vi "Actor Core.vi"(8 "error in":errorcluster, 11 "Microscope in":refnum<class "Microscope.lvclass">) -> (0 "error out":errorcluster, 3 "Actor out":refnum<class "Actor.lvclass">)   [LabVIEW 2020, in "Microscope.lvlib" / "Microscope.lvclass"]
doc: "(<B>Filename</B>: Actor Framework.lvlib:Actor.lvclass:Actor Core.vi)\n\nReceives messages to the actor, reacts to them, and initiates any error handling that may shut the actor down.\n\nDescendant classes may override this VI to append parallel tasks for the actor to complete while it handles messages. Overrides use the Call Parent Class Method node."
uses:
  Microscope.lvclass
  C:/Program Files/National Instruments/LabVIEW 2020/vi.lib/ActorFramework/Actor/Actor.lvclass
  <vilib>/ActorFramework/Actor/Actor.lvclass
  Microscope Controller/Microscope Controller.lvclass
  Microscope.lvclass/Microscope.ctl
  Device/Device/Device.lvclass
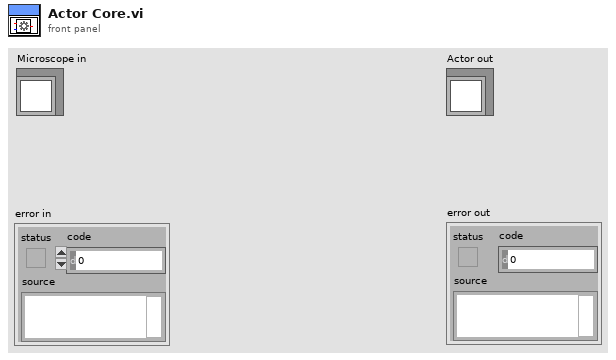
[diagram p1: front panel]
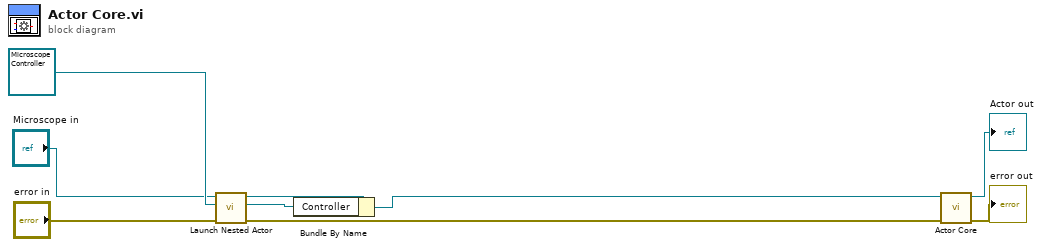
[diagram p0: block diagram]
diagram:
  n1 = call <vilib>:"Launch Nested Actor.vi"("error in (no error)"="error in", "Nested Actor"=refnum<class "Microscope Controller.lvclass"> refnum ("Microscope Controller.lvlib:Microscope Controller.lvclass"), "Caller Actor in"="Microscope in") -> ("error out"=w4:errorcluster, "Nested Actor's Enqueuer"=w1:refnum<class "Message Enqueuer.lvclass">, "Caller Actor out"=w3:refnum<class "Microscope.lvclass">)  [unwired: 6 in]
  n2 = Bundle By Name(cluster=w3, "Controller"=w1) -> (w2:refnum<class "Microscope.lvclass">)
  n3 = call-parent "Actor Core.vi"("error in"=w4, "Actor in"=w2) -> ("error out"=→"error out":errorcluster, "Actor out"=→"Actor out":refnum<class "Actor.lvclass">)  [unwired: 8 in]
